vi "Create Digital Output Module.vi"(8 "error in":errorcluster, 10 "channel settings":T1[](array[typedef]), 11 "module in":refnum<class "Module.lvclass">) -> (0 "error out":errorcluster, 3 "module out":refnum<class "Module.lvclass">)   [LabVIEW 2017, in "Scan Engine Scripting.lvlib" / "Module.lvclass"]
uses:
  Module.lvclass
  Mode Classes/Controls/digital channel settings.ctl
  Mode Classes/Digital Output Mode/Digital Output Mode.lvclass
  C:/dev/github.com/debryant/niveristand-scan-engine-ethercat-custom-device/Custom Device Source/Scripting/Modules/Mode Classes/Mode/Mode.lvclass
  Channel Classes/DO Channel/DO Channel.lvclass
  C:/dev/github.com/debryant/niveristand-scan-engine-ethercat-custom-device/Custom Device Source/Scripting/Modules/Channel Classes/Channel/Channel.lvclass
  Scan Engine Scripting.lvlib
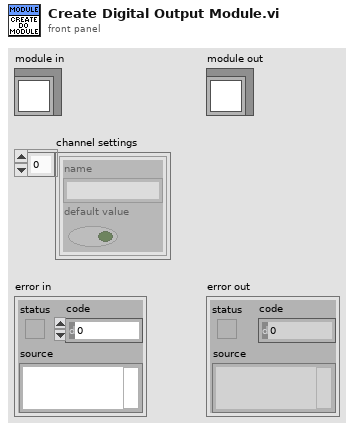
[diagram p1: front panel]
types:
  T1 = typedef "Scan Engine Scripting.lvlib/digital channel settings.ctl" = cluster{"name":string, "default value":bool}
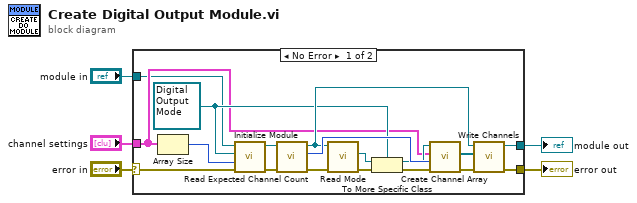
[diagram p0: block diagram]
diagram:
  n1 = case shown="No Error" "error in" {
    selector: "error in" -> [w11 w25]
    tunnel: [w10 w25] -> w4
    tunnel: [w8 w24] -> w2
    tunnel: "module in" -> [w9 w24]
    tunnel: "channel settings" -> [w12 _]
    frame No Error {
      w14 = refnum<class "Digital Output Mode.lvclass"> refnum ("Scan Engine Scripting.lvlib:Digital Output Mode.lvclass")
      n2 = Array Size(array=w12) -> (size(s)=w18:i32)
      n3 = call-dynamic "Initialize Module.vi"("error in"=w11, "channel array size"=w18, "mode"=w14, "module in"=w9) -> ("error out"=w22:errorcluster, "module out"=w23:refnum<class "Module.lvclass">)  [unwired: 6 in]
      n4 = call-dynamic "Read Expected Channel Count.vi"("error in"=w22, "module in"=w23) -> ("error out"=w16:errorcluster, "expected channel count"=w19:i32, "module out"=w17:refnum<class "Module.lvclass">)  [unwired: 7 in]
      n5 = call-dynamic "Read Mode.vi"("error in"=w16, "module in"=w17) -> ("error out"=w7:errorcluster, "mode"=w15:refnum<class "Mode.lvclass">)  [unwired: 7 in, 1 out]
      n6 = To More Specific Class(target class=w14, reference=w15, error in=w7) -> (specific class reference=w13:refnum<class "Digital Output Mode.lvclass">, error out=w6:errorcluster)
      n7 = call "Create Channel Array.vi"("error in"=w6, "expected channel count"=w19, "channel settings"=w12, "digital output mode in"=w13) -> ("error out"=w21:errorcluster, "channels"=w20:refnum<class "DO Channel.lvclass">[])  [unwired: 5 in, 1 out]
      n8 = call-dynamic "Write Channels.vi"("error in"=w21, "channels"=w20, "module in"=w17) -> ("error out"=w10:errorcluster, "module out"=w8:refnum<class "Module.lvclass">)  [unwired: 7 in]
    }
    frame Error {
    }
  }
  "error out" <- w4
  "module out" <- w2
